vi "ApplyDLP2GUIConfig_API.vi"(8 "error in (no error)":errorcluster, 10 "DLP GUI Config":path, 11 "TopLevel in":refnum<class "TopLevel.lvclass">) -> (0 "error out":errorcluster, 3 "TopLevel out":refnum<class "TopLevel.lvclass">)   [LabVIEW 2022 SP3, in "TopLevel.lvclass"]
uses:
  TopLevel.lvclass
  Typedefs/API Command Cluster.ctl
  Typedefs/API Command Enum.ctl
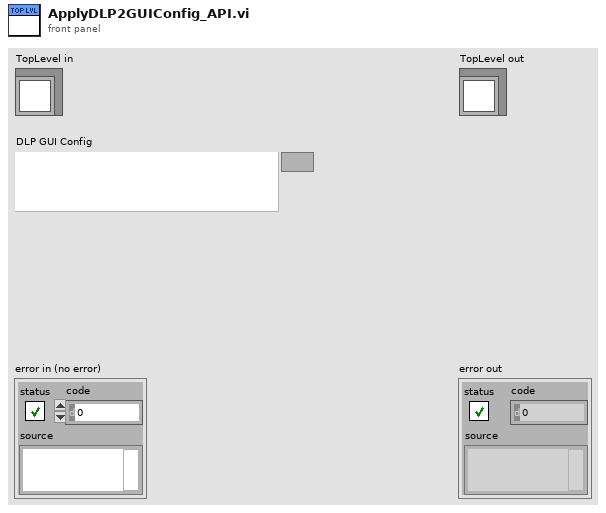
[diagram p1: front panel]
types:
  T1 = typedef "TopLevel.lvclass/API Command Enum.ctl" = enum16{"Execute Printer Commands", "Pre Purge", "Enable Ink Ch-1", "Enable Ink Ch-2", "Enable Ink Ch-3", "Enable Ink Ch-4", "Enable Ink Ch-5", "Enable Ink Ch-6", "Disable Ink Ch-1", "Disable Ink Ch-2", "Disable Ink Ch-3", "Disable Ink Ch-4", "Disable Ink Ch-5", "Disable Ink Ch-6", "ExecuteIdlePrintCycle", "StopIdlePrintCycle", "Abort", "LoadDLP2GUIConfig", "SaveDLP2GUIConfig", "PrimingMode"}
  T2 = typedef "TopLevel.lvclass/API Command Cluster.ctl" = cluster{"Command":T1, "Arguments":string, "Data":variant}
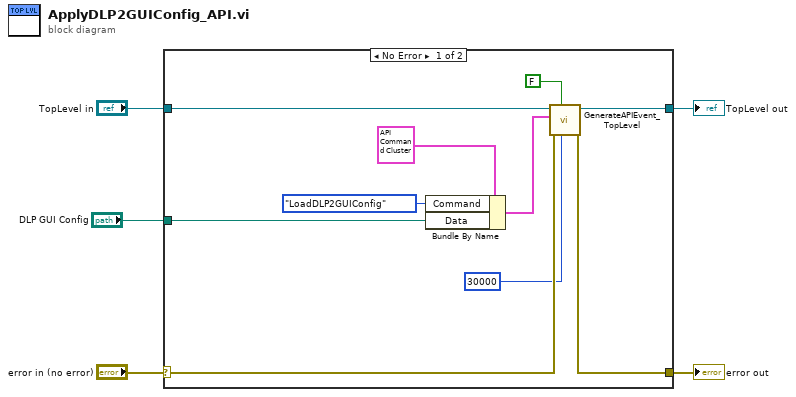
[diagram p0: block diagram]
diagram:
  n1 = case shown="No Error" "error in (no error)" {
    selector: "error in (no error)" -> [w13 w17]
    tunnel: [w12 w17] -> w4
    tunnel: [w15 w16] -> w2
    tunnel: "TopLevel in" -> [w14 w16]
    tunnel: "DLP GUI Config" -> [w6 _]
    frame No Error {
      n2 = Bundle By Name(cluster=T2 {"Command"=enum."Execute Printer Commands", "Arguments"="", "Data"=variant} ("API Command Cluster"), "Command"=API_Command_Enum."LoadDLP2GUIConfig", "Data"=w6) -> (w9:T2)
      n3 = call-dynamic "GenerateAPIEvent_TopLevel.vi"("Timeout (ms)"=u32 30000, "Wait (F)"=FALSE, "error in (no error)"=w13, "API Command Cluster"=w9, "TopLevel in"=w14) -> ("error out"=w12:errorcluster, "TopLevel out"=w15:refnum<class "TopLevel.lvclass">)  [unwired: 5 in]
    }
    frame Error {
    }
  }
  "error out" <- w4
  "TopLevel out" <- w2
